vi "DAC8568_setOutput.vi"(8 "error in (no error)":errorcluster, 9 "output":u16, 10 "channel":u8, 11 "location":u8) -> (0 "error out":errorcluster)   [LabVIEW 2015, in "ESLSCDLL.lvlib"]
uses:
  ESLSCDLL.lvlib
  Globals.vi
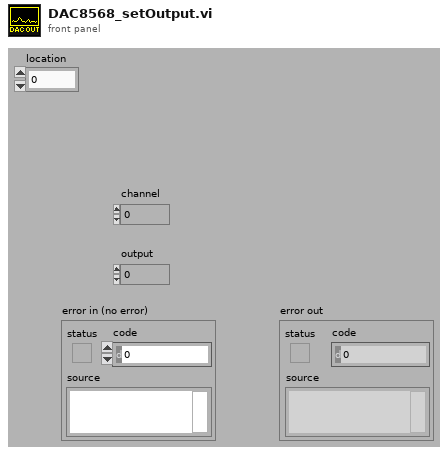
[diagram p1: front panel]
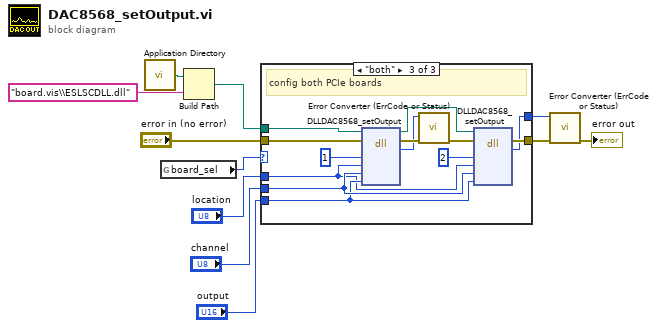
[diagram p0: block diagram]
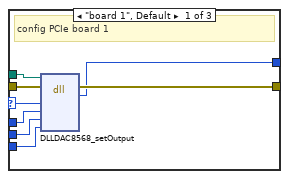
[diagram p2: hidden frame]
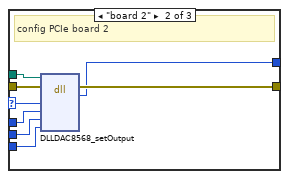
[diagram p3: hidden frame]
diagram:
  n1 = call <vilib>:"Application Directory.vi"() -> ("Application Directory"=w4:path)
  n2 = global read "Globals.vi" "board_sel"() -> (w5:enum32{"0", "board 1", "board 2", "both"})
  n3 = Build Path(base path=w4, name or relative path="board.vis\\ESLSCDLL.dll") -> (appended path=w2:path)
  n4 = case shown="\"both\"" w5 {
    selector: w5 -> [w17 w27 _]
    tunnel: "channel" -> [w19 w26 w38]
    tunnel: "output" -> [w18 w25 w37]
    tunnel: "error in (no error)" -> [w16 w24 w36]
    tunnel: [w15 w23 w32] -> w8
    tunnel: [w14 w22 w31] -> w7
    tunnel: w2 -> [w13 w21 w30]
    tunnel: "location" -> [w12 w20 w28]
    frame "board 1", Default {
      # "config PCIe board 1"
      n5 = dll-call lib="C:/ENTW/PCIE/LV64/board.vis/ESLSCDLL.dll" fn="DLLDAC8568_setOutput" ("lwlscdll.dll:DLLSetADAmpRed")(path in=w13, error in=w16, "drvno"=w17, "location"=w12, "channel"=w19, "output"=w18) -> (error out=w15:errorcluster, "es_status_codes"=w14:i32)  [unwired: 5 in, 1 out]
    }
    frame "board 2" {
      # "config PCIe board 2"
      n6 = dll-call lib="C:/ENTW/PCIE/LV64/board.vis/ESLSCDLL.dll" fn="DLLDAC8568_setOutput" ("lwlscdll.dll:DLLSetADAmpRed")(path in=w21, error in=w24, "drvno"=w27, "location"=w20, "channel"=w26, "output"=w25) -> (error out=w23:errorcluster, "es_status_codes"=w22:i32)  [unwired: 5 in, 1 out]
    }
    frame "both" {
      # "config both PCIe boards"
      n7 = dll-call lib="C:/ENTW/PCIE/LV64/board.vis/ESLSCDLL.dll" fn="DLLDAC8568_setOutput" ("lwlscdll.dll:DLLSetADAmpRed")(path in=w30, error in=w36, "drvno"=u32 1, "location"=w28, "channel"=w38, "output"=w37) -> (path out=w29:path, error out=w35:errorcluster, "es_status_codes"=w34:i32)  [unwired: 5 in]
      n8 = call "Error Converter (ErrCode or Status).vi"("error in (no error)"=w35, "error code"=w34) -> ("error out"=w33:errorcluster)  [unwired: 9 in]
      n9 = dll-call lib="C:/ENTW/PCIE/LV64/board.vis/ESLSCDLL.dll" fn="DLLDAC8568_setOutput" ("lwlscdll.dll:DLLSetADAmpRed")(path in=w29, error in=w33, "drvno"=u32 2, "location"=w28, "channel"=w38, "output"=w37) -> (error out=w32:errorcluster, "es_status_codes"=w31:i32)  [unwired: 5 in, 1 out]
    }
  }
  n10 = call "Error Converter (ErrCode or Status).vi"("error in (no error)"=w8, "error code"=w7) -> ("error out"=→"error out":errorcluster)  [unwired: 9 in]
